vi "Process Message.vi"(0 "Received Message":string) -> (1 "Message Header":string, 2 "Message Body":string)   [LabVIEW 2013]
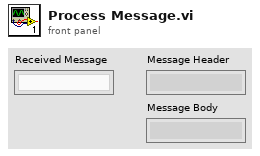
[diagram p1: front panel]
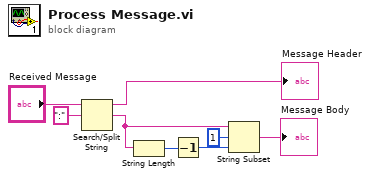
[diagram p0: block diagram]
diagram:
  n1 = Search/Split String(string="Received Message", search string/char (-)=":") -> (substring before match=→"Message Header":string, match + rest of string=w2:string)  [unwired: 1 in, 1 out]
  n2 = String Length(string=w2) -> (length=w5:i32)
  n3 = Decrement(x=w5) -> (x-1=w4:i32)
  n4 = String Subset(string=w2, offset (0)=1, length (rest)=w4) -> (substring=→"Message Body":string)
